vi "RT Main and Scoreboard.vi"() -> ()   [LabVIEW 2026]
uses:
  RT Image.ctl
  RT States.ctl
  Idle Pattern.ctl
  Score.ctl
  SideSelector.ctl
  RT Commands.ctl
  Game Settings.ctl
  2 Player Bitfile dynRef.ctl
  <vilib>/FPGAPlugInAG/cRIO-9047/niLvFpga_Open_cRIO-9047.vi
  <vilib>/rvi/interface/common/dynamic/niFpgaDynamicAddResources.vi
  <vilib>/FPGAPlugInAG/Dynamic/niLvFpga_Run_Dynamic.vi
  <vilib>/Utility/error.llb/Error Cluster From Error Code.vi
  <vilib>/rvi/errors/niLvFpgaAdjustHostInterfaceError.vi
  <vilib>/FPGAPlugInAG/Dynamic/niLvFpga_Abort_Dynamic.vi
  <vilib>/FPGAPlugInAG/Dynamic/niLvFpga_Close_Dynamic.vi
  <vilib>/rvi/interface/nirviOpenFPGA/nirviOpenFPGA.xnode
  FPGA Bitfiles/speedofvight_IdlePattern.lvbitx
  <vilib>/rvi/interface/nirviMethod/nirviMethod.xnode
  <vilib>/rvi/interface/nirviReadWriteControl/nirviReadWriteControl.xnode
  <vilib>/rvi/interface/nirviCloseFPGA/nirviCloseFPGA.xnode
  FPGA Bitfiles/speedofvight_1Player.lvbitx
  FPGA Bitfiles/speedofvight_2Player.lvbitx
  <vilib>/rvi/interface/Simulation/niFpgaSimulationCallBeginRW.vi
  NiFpgaLv.dll
  <vilib>/Utility/Data Type/NI_Data Type.lvlib
panel:
  out "error out 3":errorcluster
  out "error out 2":errorcluster
  out "x-y*floor(x/y)":u32
  out "floor(x/y)":u32
  in  "Winner Display time, ms":u32=7000
  in  "2 Players":bool
  in  "Idle Pattern Cycle Time":u32=5000
  in  "abort":bool
  in  "End Idle":bool
  out "error out":errorcluster
  in  "Speed Threshold, ticks":u64=3000
  in  "Debounce Threshold, ticks":u64=5000
  in  "Game Time":u32=4
  in  "End Game":bool
  out "Score P1":u16 format="%03.0f"
  out "Score P2":u16 format="%03.0f"
  out "2D Picture":T1
  out "Time Remaining":u32 format="%03.0f"
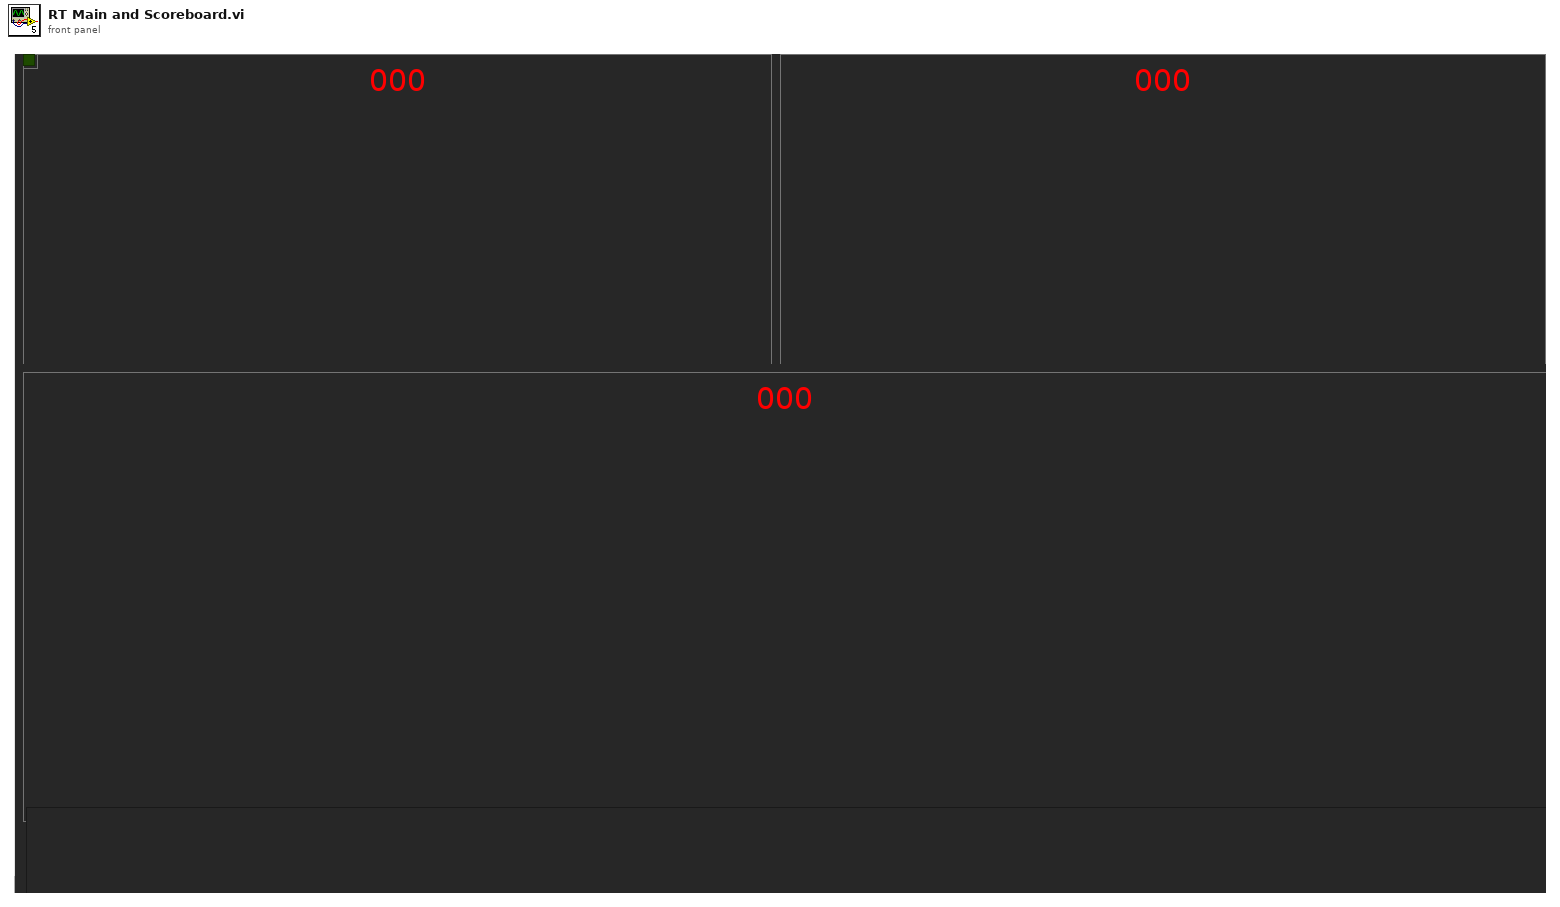
[diagram p1: front panel]
types:
  T1 = typedef "RT Image.ctl" = picture
  T2 = typedef "Score.ctl" = cluster{"Score P1":u16, "Score P2":u16, "Winner Selection":T3}
  T3 = typedef "SideSelector.ctl" = enum16{"P12", "P1", "P2"}
  T4 = cluster{"Debounce Threshold, ticks":u64, "Speed Threshold, ticks":u64, "Game Time":u32, "Idle Pattern Cycle Time, ms":u32, "Winner Display time, ms":u32, "Final Score":T2}
  T5 = typedef "Idle Pattern.ctl" = enum16{"Expanding Circle", "Plasma", "Radar Sweep", "Matrix Rain", "Campfire", "Diagonal Scan"}
  T6 = typedef "RT States.ctl" = enum16{"Idle", "Configuring", "1Player", "2Player", "Display Winner"}
  T7 = typedef "RT Commands.ctl" = enum16{"<null>", "End Idle", "Reset", "Commit Settings", "Commit Host Settings"}
  T8 = typedef "2 Player Bitfile dynRef.ctl" = refnum<k20>
  T9 = typedef "Game Settings.ctl" = cluster{"Speed Threshold, ticks":u64, "Game Time":u32, "2 Players":bool}
  T10 = cluster{"Score P1":u16, "Score P2":u16, "Winner Selection":T3}
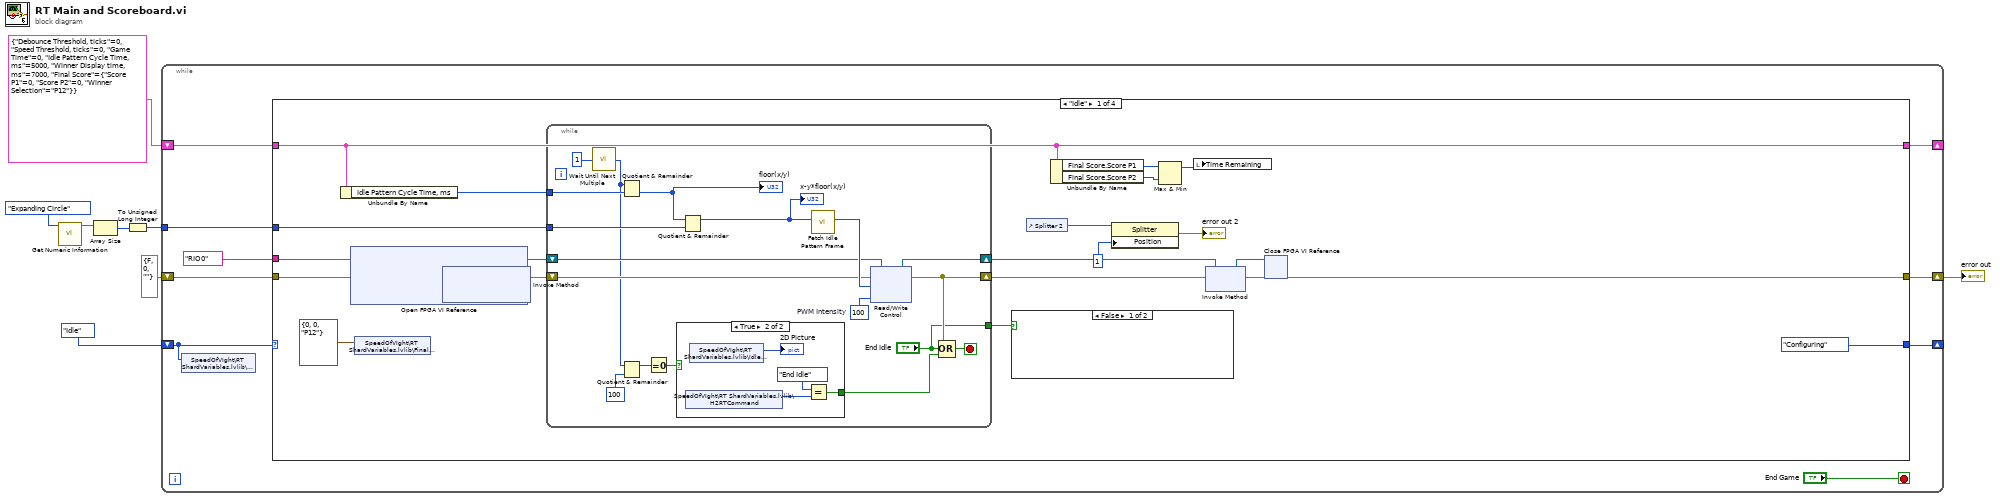
[diagram p0: block diagram]
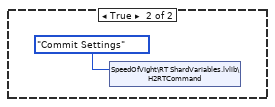
[diagram p2: hidden frame]
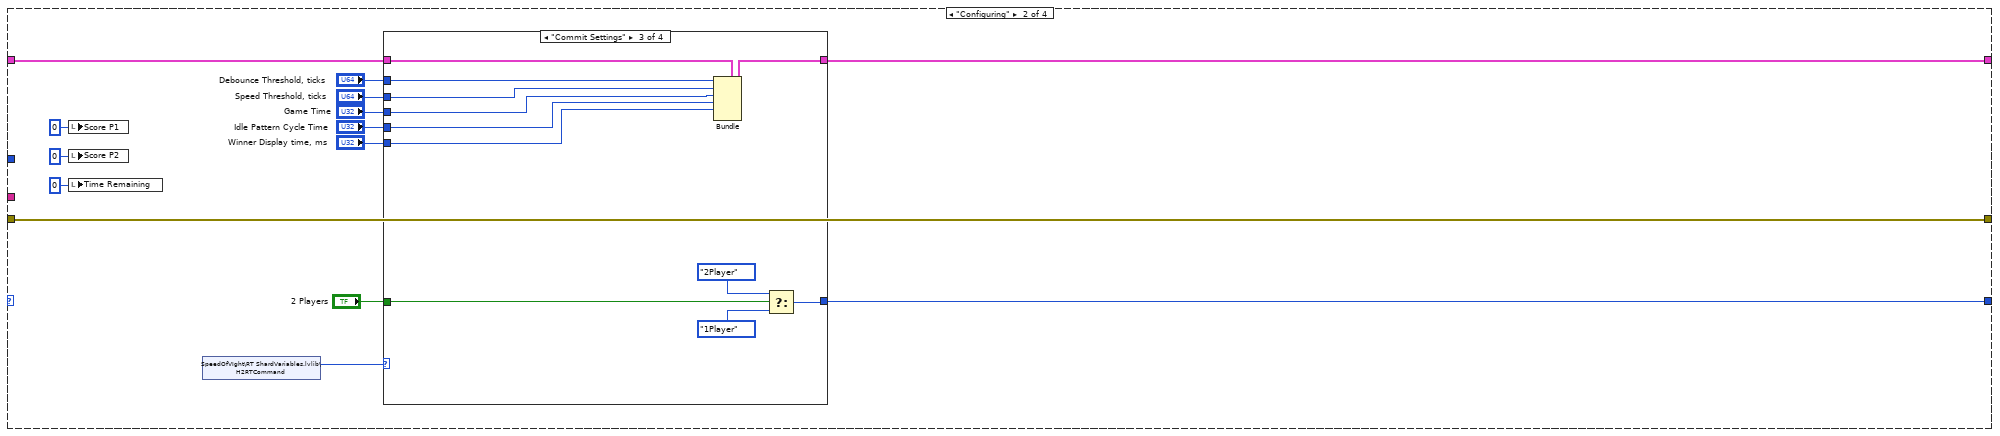
[diagram p4: hidden frame]
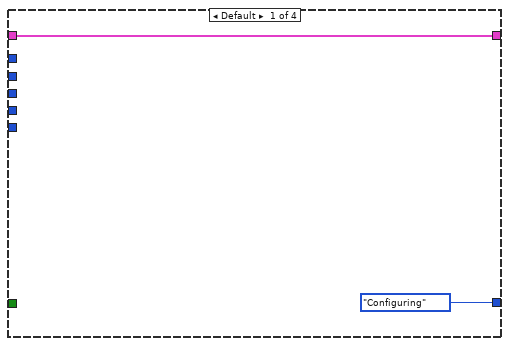
[diagram p5: hidden frame]
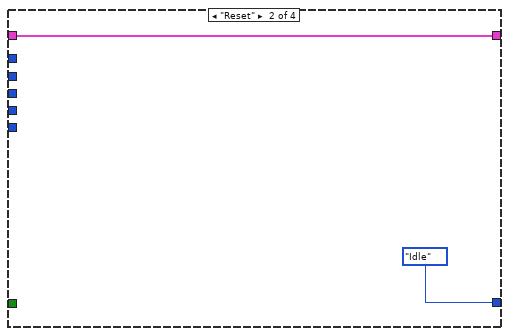
[diagram p6: hidden frame]
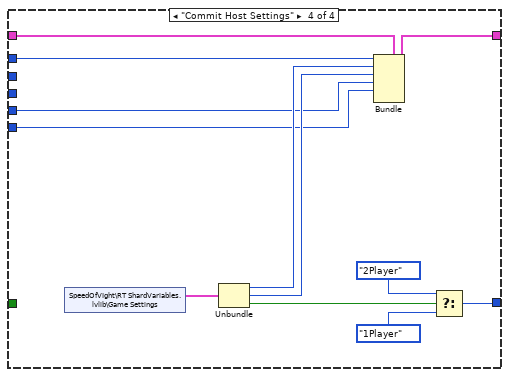
[diagram p7: hidden frame]
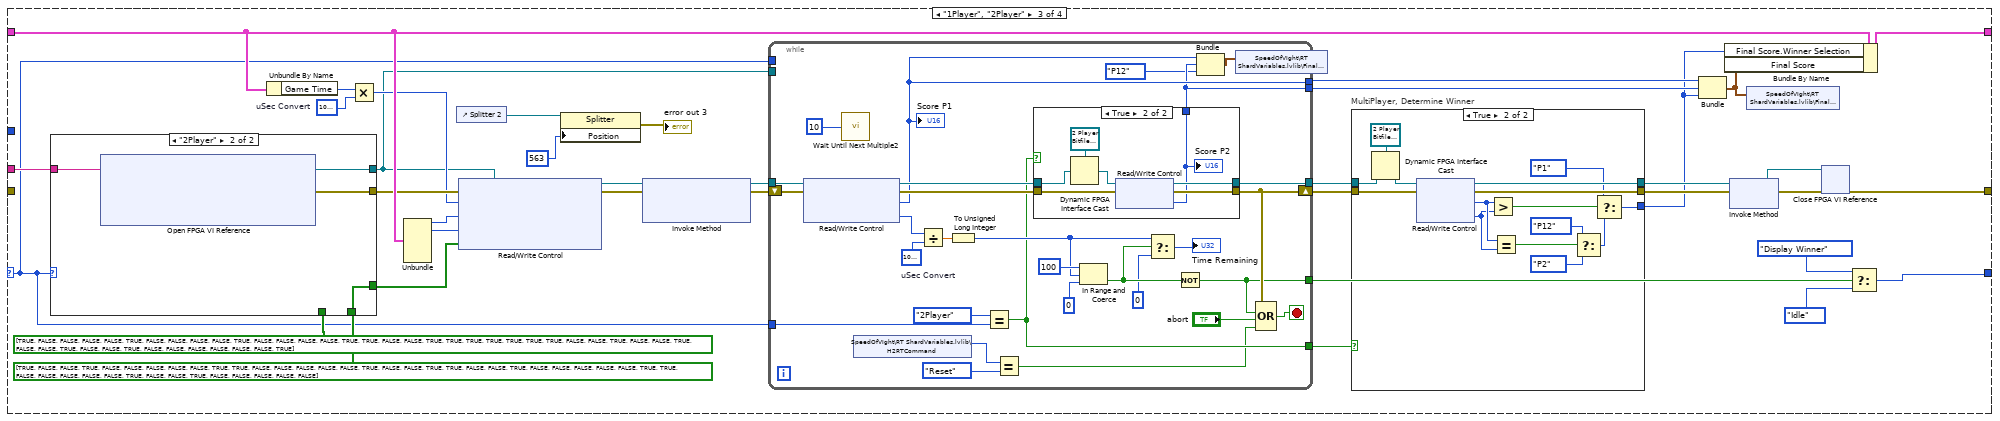
[diagram p8: hidden frame]
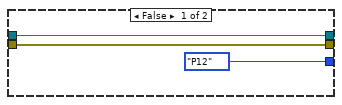
[diagram p9: hidden frame]
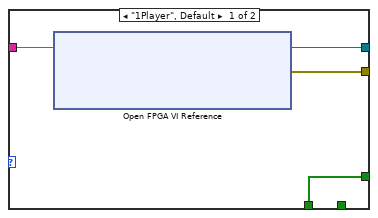
[diagram p10: hidden frame]
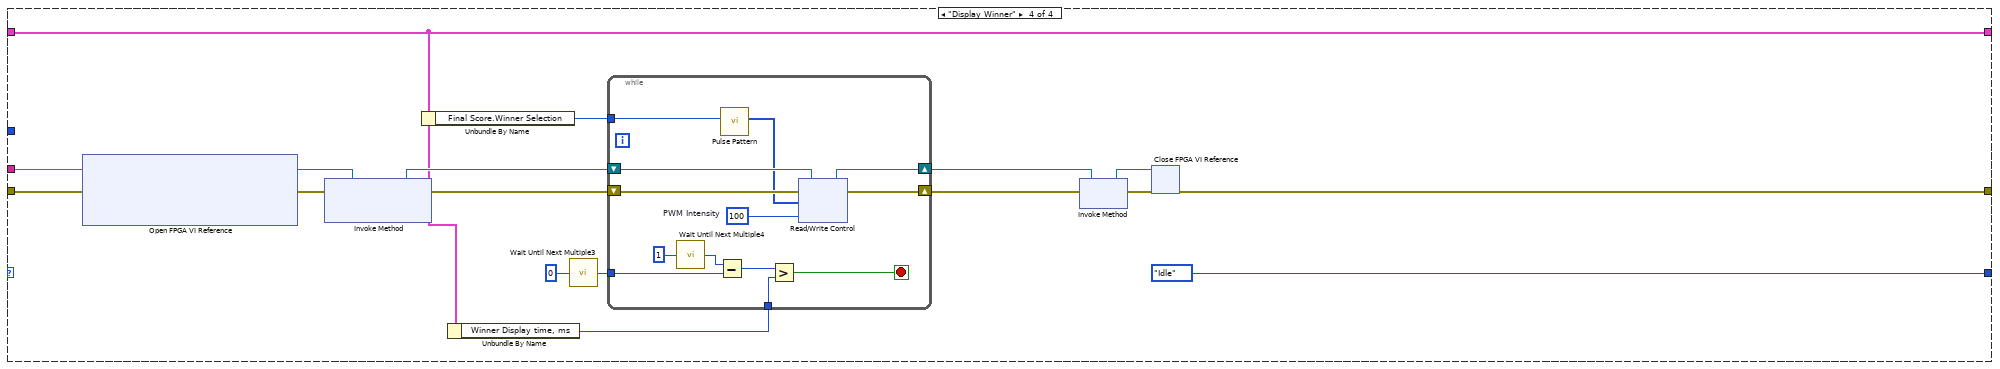
[diagram p12: hidden frame]
diagram:
  n1 = call <vilib>:"Get Numeric Information.vi"("variant"=Idle_Pattern."Expanding Circle" ("Effect")) -> ("enum names"=w6:string[])  [unwired: 7 in, 3 out]
  n2 = Array Size(array=w6) -> (size(s)=w5:i32)
  n3 = To Unsigned Long Integer(number=w5) -> (unsigned 32bit integer=w1:u32)
  n4 = while {
    shift-right: [w13] -> _
    shift-left: RT_States."Idle" ("Enum") -> [w10]
    tunnel: w1 -> [w16]
    shift-right: [w15] -> w4
    shift-left: errorcluster {"status"=FALSE, "code"=0, "source"=""} ("error out") -> [w14]
    shift-right: [w11] -> _
    shift-left: T4 {"Debounce Threshold, ticks"=0, "Speed Threshold, ticks"=0, "Game Time"=0, "Idle Pattern Cycle Time, ms"=5000, "Winner Display time, ms"=7000, "Final Score"={"Score P1"=0, "Score P2"=0, "Winner Selection"=enum."P12"}} ("cluster") -> [w12]
    stop <- "End Game" stop-if-true
    n5 = shared-variable "SpeedOfVIght\\RT ShardVariables.lvlib\\RT2HState"(w10) -> ()  [unwired: 1 in, 1 out]
    n6 = case shown="\"Idle\"" w10 {
      selector: w10 -> [_ _ w110 _]
      tunnel: tag "RIO0" ("resource name") -> [w36 _ w133 w218]
      tunnel: w16 -> [w35 _ _ _]
      tunnel: [w30 w77 w127 w213] -> w15
      tunnel: w14 -> [w29 w77 _ w212]
      tunnel: [RT_States."Configuring" ("Enum") w74 w120 RT_States."Idle" ("Enum")] -> w13
      tunnel: w12 -> [w21 w76 w141 w206]
      tunnel: [w21 w75 w121 w206] -> w11
      frame "Idle" {
        n7 = Unbundle By Name(w21) -> ("Idle Pattern Cycle Time, ms"=w27:u32)
        n8 = xnode "Open FPGA VI Reference"("error in"=w29, "resource name"=w36) -> ("FPGA VI Reference Out"=w38:refnum<k20>, "error out"=w40:errorcluster)
        n9 = shared-variable "SpeedOfVIght\\RT ShardVariables.lvlib\\Final Score"(T2 {"Score P1"=0, "Score P2"=0, "Winner Selection"=enum."P12"} ("Final Score")) -> ()  [unwired: 1 in, 1 out]
        n10 = xnode "Invoke Method"("FPGA VI Reference In"=w38, "error in"=w40) -> ("FPGA VI Reference Out"=w37:refnum<k20>, "error out"=w39:errorcluster)  [unwired: 1 in]
        n11 = while {
          shift-right: [w51] -> w32
          shift-left: w39 -> [w57]
          shift-right: [w55] -> w31
          shift-left: w37 -> [w56]
          tunnel: w35 -> [w49]
          tunnel: w27 -> [w50]
          tunnel: ["End Idle"] -> w26
          stop <- w53 stop-if-true
          w58 = u16 100  # PWM Intensity
          n12 = call "Wait Until Next Multiple"("Count(mSec)"=u32 1 ("Count(Ticks)")) -> ("Tick Count(mSec)"=w44:u32)
          n13 = Quotient & Remainder(x=w44, y=w50) -> (floor(x/y)=w48:u32)  [unwired: 1 out]
          "floor(x/y)" <- w48
          n14 = Quotient & Remainder(x=w44, y=u32 100) -> (x-y*floor(x/y)=w42:u32)  [unwired: 1 out]
          n15 = Equal To 0?(x=w42) -> (x = 0?=w45:bool)
          n16 = case shown="True" w45 {
            tunnel: [_ w62] -> w52
            frame False {
            }
            frame True {
              n17 = shared-variable "SpeedOfVIght\\RT ShardVariables.lvlib\\H2RTCommand"() -> (w61:T7)  [unwired: 1 in, 1 out]
              n18 = shared-variable "SpeedOfVIght\\RT ShardVariables.lvlib\\Idle Image"() -> (→"2D Picture":T1)  [unwired: 1 in, 1 out]
              n19 = Equal?(x=RT_Commands."End Idle", y=w61) -> (x = y?=w62:bool)
            }
          }
          n20 = Quotient & Remainder(x=w48, y=w49) -> (x-y*floor(x/y)=w47:u32)  [unwired: 1 out]
          "x-y*floor(x/y)" <- w47
          n21 = call "Fetch Idle Pattern Frame.vi"("Effect"=w47) -> ("Array"=w59:u16[])  [unwired: 10 in]
          n22 = xnode "Read/Write Control"("FPGA VI Reference In"=w56, "error in"=w57, "x"=w59, "Period"=w58) -> ("FPGA VI Reference Out"=w55:refnum<k20>, "error out"=w51:errorcluster)
          n23 = Compound Arithmetic op=OR(w51, "End Idle", w52) -> (w53:bool)
        }
        n24 = case shown="False" w26 {
          frame False {
          }
          frame True {
            n25 = shared-variable "SpeedOfVIght\\RT ShardVariables.lvlib\\H2RTCommand"(RT_Commands."Commit Settings" ("H2RTCommand")) -> ()  [unwired: 1 in, 1 out]
          }
        }
        n26 = control-ref of="Splitter 2"() -> (w24:refnum<vi>)
        n27 = Unbundle By Name(w21) -> ("Final Score.Score P1"=w20:u16, "Final Score.Score P2"=w19:u16)
        n28 = property class="Splitter"(reference=w24, "Position"=1 ("Splitter Position")) -> (error out=→"error out 2":errorcluster)  [unwired: 1 in, 1 out]
        n29 = Max & Min(x=w20, y=w19) -> (max(x,y)=w18:u16)  [unwired: 1 out]
        n30 = local write "Time Remaining"(w18) -> ()
        n31 = xnode "Invoke Method"("FPGA VI Reference In"=w31, "error in"=w32) -> ("FPGA VI Reference Out"=w34:refnum<k20>, "error out"=w33:errorcluster)
        n32 = xnode "Close FPGA VI Reference"("FPGA VI Reference In"=w34, "error in"=w33) -> ("error out"=w30:errorcluster)
      }
      frame "Configuring" {
        n33 = local write "Score P1"(u16 0 ("Score P1")) -> ()
        n34 = local write "Score P2"(u16 0 ("Score P2")) -> ()
        n35 = local write "Time Remaining"(u32 0 ("Time Remaining")) -> ()
        n36 = shared-variable "SpeedOfVIght\\RT ShardVariables.lvlib\\H2RTCommand"() -> (w70:T7)  [unwired: 1 in, 1 out]
        n37 = case shown="\"Commit Settings\"" w70 {
          tunnel: w76 -> [w78 w81 w90 w102]
          tunnel: [w78 w81 w89 w101] -> w75
          tunnel: [RT_States."Configuring" ("Enum") RT_States."Idle" ("Enum") w88 w100] -> w74
          tunnel: "Winner Display time, ms" -> [_ _ w82 w93]
          tunnel: "Idle Pattern Cycle Time" -> [_ _ w83 w94]
          tunnel: "Speed Threshold, ticks" -> [_ _ w87 _]
          tunnel: "Debounce Threshold, ticks" -> [_ _ w86 w99]
          tunnel: "Game Time" -> [_ _ w85 _]
          tunnel: "2 Players" -> [_ _ w84 _]
          frame Default {
          }
          frame "Reset" {
          }
          frame "Commit Settings" {
            n38 = Bundle(cluster=w90, "Debounce Threshold, ticks"=w86, "Speed Threshold, ticks"=w87, "Game Time"=w85, "Idle Pattern Cycle Time, ms"=w83, "Winner Display time, ms"=w82) -> (w89:T4)  [unwired: 1 in]
            n39 = Select(t=RT_States."2Player" ("Enum"), s=w84, f=RT_States."1Player" ("Enum")) -> (s? t:f=w88:T6)
          }
          frame "Commit Host Settings" {
            n40 = shared-variable "SpeedOfVIght\\RT ShardVariables.lvlib\\Game Settings"() -> (w98:T9)  [unwired: 1 in, 1 out]
            n41 = Unbundle(w98) -> ("Speed Threshold, ticks"=w97:u64, "Game Time"=w95:u32, "2 Players"=w96:bool)
            n42 = Bundle(cluster=w102, "Debounce Threshold, ticks"=w99, "Speed Threshold, ticks"=w97, "Game Time"=w95, "Idle Pattern Cycle Time, ms"=w94, "Winner Display time, ms"=w93) -> (w101:T4)  [unwired: 1 in]
            n43 = Select(t=RT_States."2Player" ("Enum"), s=w96, f=RT_States."1Player" ("Enum")) -> (s? t:f=w100:T6)
          }
        }
      }
      frame "1Player", "2Player" {
        w140 = u32 1000000  # uSec Convert
        n44 = case shown="\"2Player\"" w110 {
          tunnel: [w163 w167] -> w137
          tunnel: [w162 w166] -> w109
          tunnel: w133 -> [w161 w165]
          tunnel: [w160 w164] -> w108
          tunnel: bool[] [TRUE, FALSE, FALSE, TRUE, FALSE, FALSE, FALSE, FALSE, FALSE, TRUE, TRUE, FALSE, FALSE, FALSE, FALSE, FALSE, TRUE, FALSE, FALSE, TRUE, TRUE, FALSE, FALSE, TRUE, FALSE, FALSE, FALSE, FALSE, FALSE, TRUE, TRUE, FALSE, FALSE, FALSE, FALSE, FALSE, TRUE, FALSE, FALSE, TRUE, FALSE, FALSE, FALSE, FALSE, FALSE] ("appended array") -> [_ w164]
          tunnel: bool[] [TRUE, FALSE, FALSE, FALSE, FALSE, TRUE, FALSE, FALSE, FALSE, FALSE, TRUE, FALSE, FALSE, FALSE, FALSE, TRUE, TRUE, FALSE, FALSE, TRUE, TRUE, TRUE, TRUE, TRUE, TRUE, TRUE, FALSE, FALSE, TRUE, FALSE, FALSE, TRUE, FALSE, FALSE, TRUE, FALSE, FALSE, TRUE, FALSE, FALSE, FALSE, FALSE, FALSE, FALSE, TRUE] ("appended array") -> [w160 _]
          frame "1Player", Default {
            n45 = xnode "Open FPGA VI Reference"("resource name"=w161) -> ("FPGA VI Reference Out"=w162:refnum<k20>, "error out"=w163:errorcluster)  [unwired: 1 in]
          }
          frame "2Player" {
            n46 = xnode "Open FPGA VI Reference"("resource name"=w165) -> ("FPGA VI Reference Out"=w166:refnum<k20>, "error out"=w167:errorcluster)  [unwired: 1 in]
          }
        }
        n47 = Unbundle By Name(w141) -> ("Game Time"=w130:u32)
        n48 = Multiply(x=w130, y=w140) -> (x*y=w134:u32)
        n49 = Unbundle(w141) -> ("Debounce Threshold, ticks"=w132:u64, "Speed Threshold, ticks"=w131:u64)  [unwired: 4 out]
        n50 = control-ref of="Splitter 2"() -> (w107:refnum<vi>)
        n51 = xnode "Read/Write Control"("FPGA VI Reference In"=w109, "error in"=w137, "Game Time, uS"=w134, "Debounce Threshold, ticks"=w132, "Speed Threshold, ticks"=w131, "Starting Lights"=w108) -> ("FPGA VI Reference Out"=w135:refnum<k20>, "error out"=w136:errorcluster)
        n52 = property class="Splitter"(reference=w107, "Position"=563 ("Splitter Position")) -> (error out=→"error out 3":errorcluster)  [unwired: 1 in, 1 out]
        n53 = xnode "Invoke Method"("FPGA VI Reference In"=w135, "error in"=w136) -> ("FPGA VI Reference Out"=w139:refnum<k20>, "error out"=w138:errorcluster)  [unwired: 1 in]
        n54 = while {
          tunnel: w139 -> [w196]
          shift-right: [w189] -> w124
          shift-left: w138 -> [w195]
          tunnel: w110 -> [w187]
          tunnel: [w183] -> w125
          tunnel: [w176] -> w118
          tunnel: [w175] -> w126
          tunnel: [w171] -> w114
          tunnel: [w170] -> w113
          tunnel: w110 -> [_]
          tunnel: w109 -> [_]
          stop <- w190 stop-if-true
          w193 = u32 1000000  # uSec Convert
          n55 = xnode "Read/Write Control"("FPGA VI Reference In"=w196, "error in"=w195) -> ("FPGA VI Reference Out"=w188:refnum<k20>, "error out"=w191:errorcluster, "Score P1"=w171:u16, "Time Remaining"=w180:u32)
          "Score P1" <- w171
          n56 = call "Wait Until Next Multiple2"("Count(mSec)"=u32 10 ("Count(Ticks)")) -> ()  [unwired: 1 out]
          n57 = shared-variable "SpeedOfVIght\\RT ShardVariables.lvlib\\H2RTCommand"() -> (w172:T7)  [unwired: 1 in, 1 out]
          n58 = Divide(x=w180, y=w193) -> (x/y=w194:dbl)
          n59 = To Unsigned Long Integer(number=w194) -> (unsigned 32bit integer=w177:u32)
          n60 = Equal?(x=RT_States."2Player", y=w187) -> (x = y?=w175:bool)
          n61 = Equal?(x=w172, y=RT_Commands."Reset") -> (x = y?=w173:bool)
          n62 = case shown="True" w175 {
            tunnel: w191 -> [w198 w205]
            tunnel: [w198 w204] -> w189
            tunnel: w188 -> [w197 w202]
            tunnel: [w197 w200] -> w183
            tunnel: [_ w199] -> w170
            frame False {
            }
            frame True {
              n63 = Dynamic FPGA Interface Cast(Session In=T8 refnum ("FPGA Interface"), Type=w202) -> (Session Out=w201:T8)
              n64 = xnode "Read/Write Control"("FPGA VI Reference In"=w201, "error in"=w205) -> ("FPGA VI Reference Out"=w200:T8, "error out"=w204:errorcluster, "Score P2"=w199:u16)
              "Score P2" <- w199
            }
          }
          n65 = In Range and Coerce(upper limit=u32 100, x=w177, lower limit=u32 0 ("y")) -> (In Range?=w181:bool)  [unwired: 1 out]
          n66 = Select(t=w177, s=w181, f=u32 0 ("y")) -> (s? t:f=→"Time Remaining":u32)
          n67 = Not(x=w181) -> (.not. x?=w176:bool)
          n68 = Bundle("Score P1"=w171, "Score P2"=w170, "Winner Selection"=SideSelector."P12") -> (w168:T10)  [unwired: 1 in]
          n69 = shared-variable "SpeedOfVIght\\RT ShardVariables.lvlib\\Final Score"(w168) -> ()  [unwired: 1 in, 1 out]
          n70 = Compound Arithmetic op=OR(w189, w176, "abort", w173) -> (w190:bool)
        }
        n71 = case "MultiPlayer, Determine Winner" shown="True" w126 {
          tunnel: w125 -> [w143 w155]
          tunnel: w124 -> [w144 w159]
          tunnel: [w144 w158] -> w123
          tunnel: [w143 w157] -> w122
          tunnel: [SideSelector."P12" ("Winner Selection") w150] -> w111
          frame False {
          }
          frame True {
            n72 = Dynamic FPGA Interface Cast(Session In=T8 refnum ("FPGA Interface"), Type=w155) -> (Session Out=w156:T8)
            n73 = xnode "Read/Write Control"("FPGA VI Reference In"=w156, "error in"=w159) -> ("FPGA VI Reference Out"=w157:T8, "error out"=w158:errorcluster, "Score P1"=w153:u16, "Score P2"=w149:u16)
            n74 = Greater?(x=w153, y=w149) -> (0:w154:bool)
            n75 = Equal?(x=w153, y=w149) -> (x = y?=w152:bool)
            n76 = Select(t=SideSelector."P12" ("Winner Selection"), s=w152, f=SideSelector."P2" ("Winner Selection")) -> (s? t:f=w146:T3)
            n77 = Select(t=SideSelector."P1" ("Winner Selection"), s=w154, f=w146) -> (s? t:f=w150:T3)
          }
        }
        n78 = Bundle("Score P1"=w114, "Score P2"=w113, "Winner Selection"=w111) -> (w112:T10)  [unwired: 1 in]
        n79 = Bundle By Name(cluster=w141, "Final Score.Winner Selection"=w111, "Final Score"=w112) -> (w121:T4)
        n80 = xnode "Invoke Method"("FPGA VI Reference In"=w122, "error in"=w123) -> ("FPGA VI Reference Out"=w129:refnum<k20>, "error out"=w128:errorcluster)
        n81 = shared-variable "SpeedOfVIght\\RT ShardVariables.lvlib\\Final Score"(w112) -> ()  [unwired: 1 in, 1 out]
        n82 = xnode "Close FPGA VI Reference"("FPGA VI Reference In"=w129, "error in"=w128) -> ("error out"=w127:errorcluster)
        n83 = Select(t=RT_States."Display Winner" ("Enum"), s=w118, f=RT_States."Idle" ("Enum")) -> (s? t:f=w120:T6)
      }
      frame "Display Winner" {
        n84 = xnode "Open FPGA VI Reference"("error in"=w212, "resource name"=w218) -> ("FPGA VI Reference Out"=w220:refnum<k20>, "error out"=w222:errorcluster)
        n85 = xnode "Invoke Method"("FPGA VI Reference In"=w220, "error in"=w222) -> ("FPGA VI Reference Out"=w219:refnum<k20>, "error out"=w221:errorcluster)  [unwired: 1 in]
        n86 = Unbundle By Name(w206) -> ("Final Score.Winner Selection"=w210:T3)
        n87 = Unbundle By Name(w206) -> ("Winner Display time, ms"=w207:u32)
        n88 = call "Wait Until Next Multiple3"("Count(mSec)"=u32 0 ("Count(Ticks)")) -> ("Tick Count(mSec)"=w208:u32)
        n89 = while {
          shift-right: [w235] -> w215
          shift-left: w221 -> [w233]
          shift-right: [w231] -> w214
          shift-left: w219 -> [w232]
          tunnel: w210 -> [w230]
          tunnel: w208 -> [w226]
          tunnel: w207 -> [w224]
          stop <- w223 stop-if-true
          w234 = u16 100  # PWM Intensity
          n90 = call "Wait Until Next Multiple4"("Count(mSec)"=u32 1 ("Count(Ticks)")) -> ("Tick Count(mSec)"=w227:u32)
          n91 = Subtract(x=w227, y=w226) -> (x-y=w225:u32)
          n92 = call "Pulse Pattern.vi"("Selector"=w230) -> ("Array"=w229:u16[])  [unwired: 10 in]
          n93 = Greater?(x=w225, y=w224) -> (0:w223:bool)
          n94 = xnode "Read/Write Control"("FPGA VI Reference In"=w232, "error in"=w233, "x"=w229, "Period"=w234) -> ("FPGA VI Reference Out"=w231:refnum<k20>, "error out"=w235:errorcluster)
        }
        n95 = xnode "Invoke Method"("FPGA VI Reference In"=w214, "error in"=w215) -> ("FPGA VI Reference Out"=w217:refnum<k20>, "error out"=w216:errorcluster)
        n96 = xnode "Close FPGA VI Reference"("FPGA VI Reference In"=w217, "error in"=w216) -> ("error out"=w213:errorcluster)
      }
    }
  }
  "error out" <- w4
